vi "Chroma 1905x Series Preset AGC.vi"(8 "error in (no error)":errorcluster, 10 "AGC":u16(ring) items=["OFF", "ON"], 11 "VISA resource name":refnum<visa-resource-name>) -> (0 "error out":errorcluster, 3 "VISA resource name out":refnum<visa-resource-name>)   [LabVIEW 2025]
doc: "Contact Chroma\nTEL: +886-2-2298-3855 \nTEL: +886-3-397-5788 \nFAX: +886-2-2298-3596\nFAX: +886-3-327-4703 \nURL: http://www.chromaate.com \nE-mail: chroma@chroma.com.tw"
panel:
  # "Automatic Gain Control"
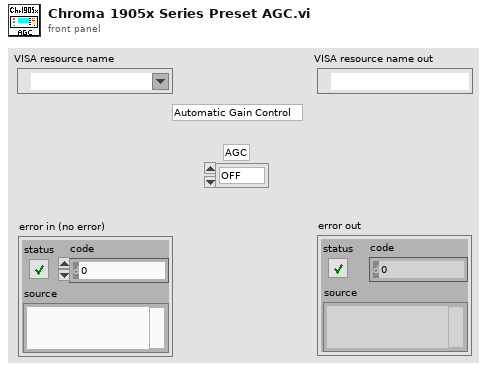
[diagram p1: front panel]
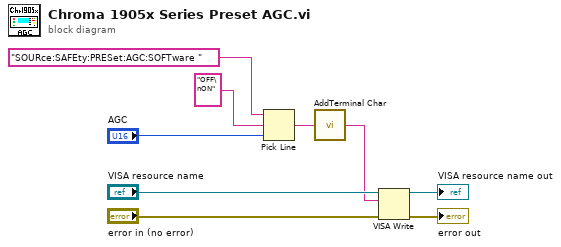
[diagram p0: block diagram]
diagram:
  n1 = Pick Line(string ("")="SOURce:SAFEty:PRESet:AGC:SOFTware ", multi-line string="OFF\nON", line index="AGC") -> (output string=w6:string)
  n2 = call "AddTerminal Char.vi"("Cmd string"=w6) -> ("Concatenated String"=w1:string)  [unwired: 4 in]
  n3 = VISA Write(VISA resource name="VISA resource name", write buffer=w1, error in (no error)="error in (no error)") -> (VISA resource name out=→"VISA resource name out":refnum<visa-resource-name>, error out=→"error out":errorcluster)  [unwired: 1 out]
